vi "Main_SCADA.vi"() -> ()   [LabVIEW 2022 SP3]
uses:
  <vilib>/Instr/_visa.llb/VISA Configure Serial Port (Instr).vi
  <vilib>/Utility/file.llb/Write Delimited Spreadsheet (string).vi
panel:
  out "Erreur VISA":errorcluster
  out "JAUGE MENACE 1-5":dbl(knob)=3.0 scale=1.0..5.0
  in  "Seuil CRC":dbl=8.0
  in  "IDS actif":bool=TRUE
  in  "Seuil variation":dbl=1.0
  in  "Nombre de cycles":dbl=5.0
  out "THREAT LEVEL":dbl=3.0
  out "Dernier snapshot":path
  out "FORENSIC SNAPSHOT TRIGGERED":bool
  in  "Baud rate":u32=115200
  in  "Port COM":refnum<visa-resource-name>="COM10"
  out "Trame recue":string
  out "CRC valides":i16
  in  "Fichier log":path=path "C:/Users/Frankel/Documents/Cours L3/Les réseaux industriels ICS et SCADA/Tp/Projet_Centrifugeuse_ICS/Data/logs.csv"
  out "Connected":bool
  out "COMMUNICATION":string="Disconnected"
  out "CRC invalides":i16=11
  out "SIGNAL FREEZE DETECTED":bool
  out "CRC VALID":bool
  out "RPM":i32
  out "STATE":string
  in  "Dossier Forensics":path=path "C:/Users/Frankel/Documents/Cours L3/Les réseaux industriels ICS et SCADA/Tp/Projet_Centrifugeuse_ICS/Forensics"
  in  "STOP":bool
  # "SCADA / IDS - CENTRIFUGEUSE - Banc de test ICS (laboratoire isole, trames recues de l Arduino par liaison serie)"
  # "SYNOPTIQUE :   [ PLC Arduino ]  -->  [ L298N + Moteur ]  -->  [ Mesure RPM (capteur IR) ]  -->  [ SCADA + IDS LabVIEW ]        PIR = detection d acces physique"
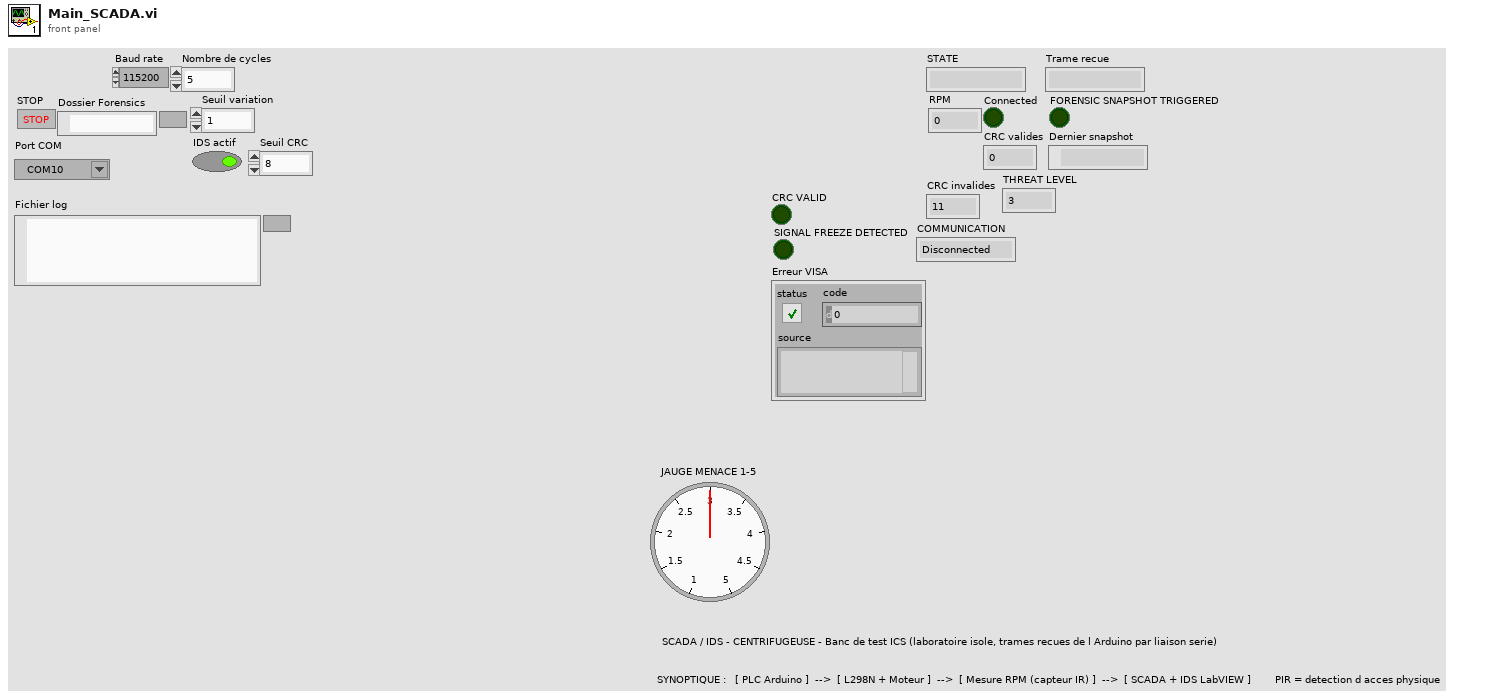
[diagram p1: front panel]
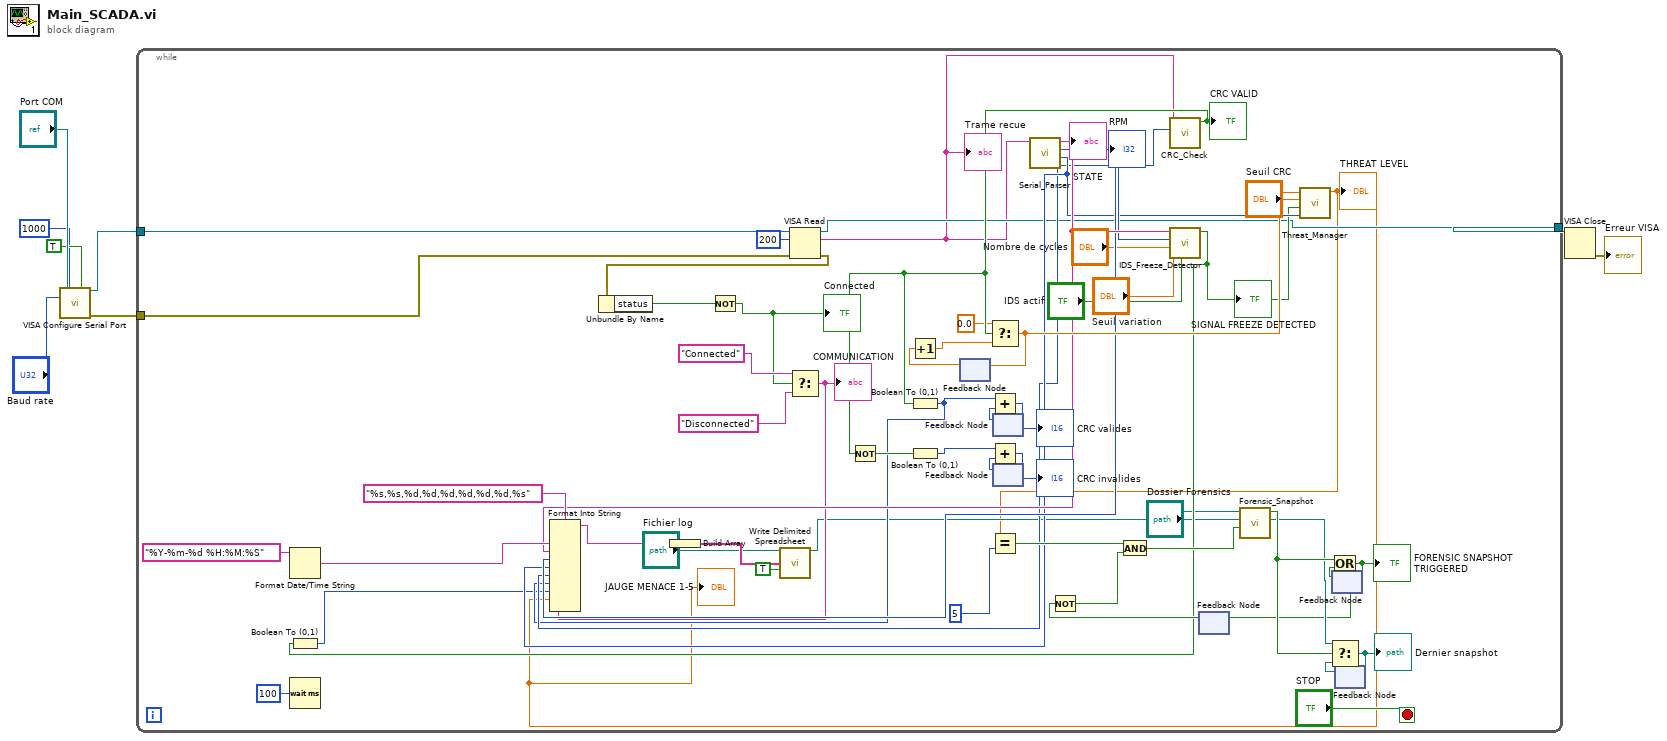
[diagram p0: block diagram]
diagram:
  n1 = call-poly "VISA Configure Serial Port"("VISA resource name"="Port COM", "timeout (10sec)"=u32 1000, "Enable Termination\nChar (T)"=TRUE ("Enable Termination\nChar (T)"), "baud rate (9600)"="Baud rate") -> ("VISA resource name out"=w8:refnum<visa-resource-name>, "error out"=w7:errorcluster)  [unwired: 10 in]
  n2 = while {
    tunnel: w8 -> [w21]
    tunnel: w7 -> [w20]
    tunnel: [w19] -> w6
    stop <- "STOP" stop-if-true
    n3 = Format Date/Time String(time format string (%c)="%Y-%m-%d %H:%M:%S") -> (date/time string=w37:string)  [unwired: 2 in]
    n4 = Wait (ms)(milliseconds to wait=u32 100) -> ()  [unwired: 1 out]
    n5 = VISA Read(VISA resource name=w21, byte count=u32 200, error in (no error)=w20) -> (VISA resource name out=w19:refnum<visa-resource-name>, read buffer=w10:string, error out=w45:errorcluster)  [unwired: 1 out]
    "Trame recue" <- w10
    n6 = Unbundle By Name(w45) -> ("status"=w42:bool)
    n7 = Not(x=w42) -> (.not. x?=w9:bool)
    "Connected" <- w9
    n8 = Select(t="Connected", s=w9, f="Disconnected") -> (s? t:f=w29:string)
    "COMMUNICATION" <- w29
    n9 = feedback #1() -> (w63:dbl)  [unwired: 1 in]
    n10 = Increment(x=w63) -> (x+1=w64:dbl)
    n11 = feedback #2() -> (w61:i16)  [unwired: 1 in]
    n12 = feedback #3() -> (w57:i16)  [unwired: 1 in]
    n13 = call "Serial_Parser.vi"("Trame"=w10) -> ("CRC"=w33:i32, "PIR"=w34:i32, "RPM"=w35:i32, "STATE"=w36:string)  [unwired: 6 in, 1 out]
    "STATE" <- w36
    "RPM" <- w35
    n14 = call "CRC_Check.vi"("CRC recu"=w33, "Trame"=w10) -> ("CRC valide"=w56:bool)  [unwired: 9 in]
    "CRC VALID" <- w56
    n15 = Not(x=w56) -> (.not. x?=w60:bool)
    n16 = Boolean To (0,1)(Boolean=w56) -> (0, 1=w32:i16)
    n17 = Boolean To (0,1)(Boolean=w60) -> (0, 1=w59:i16)
    n18 = Select(t=0.0, s=w56, f=w64) -> (s? t:f=w54:dbl)
    n19 = feedback-in #1(w54) -> ()
    n20 = Add(x=w32, y=w61) -> (x+y=w62:i16)
    "CRC valides" <- w62
    n21 = Add(x=w59, y=w57) -> (x+y=w58:i16)
    "CRC invalides" <- w58
    n22 = feedback-in #2(w62) -> ()
    n23 = feedback-in #3(w58) -> ()
    n24 = call "IDS_Freeze_Detector.vi"("IDS actif"="IDS actif", "Seuil variation"="Seuil variation", "Nombre de cycles"="Nombre de cycles", "RPM"=w35, "STATE"=w36) -> ("Freeze detecte"=w30:bool)  [unwired: 6 in]
    "SIGNAL FREEZE DETECTED" <- w30
    n25 = Boolean To (0,1)(Boolean=w30) -> (0, 1=w31:i16)
    n26 = feedback #4() -> (w43:bool)  [unwired: 1 in]
    n27 = Not(x=w43) -> (.not. x?=w52:bool)
    n28 = call "Threat_Manager.vi"("PIR"=w34, "Freeze"=w30, "Seuil CRC"="Seuil CRC", "Nb CRC invalides"=w54) -> ("Threat Level"=w11:dbl)  [unwired: 7 in]
    "THREAT LEVEL" <- w11
    "JAUGE MENACE 1-5" <- w11
    n29 = Format Into String(format string="%s,%s,%d,%d,%d,%d,%d,%d,%s", w37, w36, w35, w34, w33, w32, w31, w11, w29) -> (resulting string=w27:string)  [unwired: 2 in, 1 out]
    n30 = Build Array(w27) -> (w26:string[])
    n31 = call-poly <vilib>:"Write Delimited Spreadsheet.vi"("file path (dialog if empty)"="Fichier log", "1D data"=w26, "append to file? (new file:F)"=TRUE) -> ("new file path (Not A Path if cancelled)"=w28:path)  [unwired: 11 in, 1 out]
    n32 = Equal?(x=w11, y=5) -> (x = y?=w53:bool)
    n33 = And(x=w53, y=w52) -> (x .and. y?=w51:bool)
    n34 = call "Forensic_Snapshot.vi"("Declencher"=w51, "Dossier Forensics"="Dossier Forensics", "Fichier log"=w28) -> ("Chemin snapshot"=w48:path, "Snapshot cree"=w49:bool)  [unwired: 7 in]
    n35 = feedback #5() -> (w50:bool)  [unwired: 1 in]
    n36 = Or(x=w49, y=w50) -> (x .or. y?=w44:bool)
    "FORENSIC SNAPSHOT TRIGGERED" <- w44
    n37 = feedback-in #4(w44) -> ()
    n38 = feedback-in #5(w44) -> ()
    n39 = feedback #6() -> (w46:path)  [unwired: 1 in]
    n40 = Select(t=w48, s=w49, f=w46) -> (s? t:f=w47:path)
    "Dernier snapshot" <- w47
    n41 = feedback-in #6(w47) -> ()
  }
  n42 = VISA Close(VISA resource name=w6) -> (error out=→"Erreur VISA":errorcluster)  [unwired: 1 in]
